vi "CSM - Remove Module in Broadcast Registry.vi"(0 "CSM Name":string, 11 "Error In":errorcluster caption="error in (no error)") -> (4 "CSM Name (Dup)":string, 15 "error out":errorcluster)   [LabVIEW 2017, in "Communicable State Machine.lvlib"]
doc: "### CSM - Remove Module in Broadcast Registry.vi\n\n-- <b>Controls</b> --\n- <b>CSM Name</b>:\n\n-- <b>Indicators</b> --\n- <b>CSM Name(dup)</b>:"
uses:
  _Support/FGV-BroadcastRegistry/Operation-BroadcastRegistry.ctl
  Communicable State Machine.lvlib
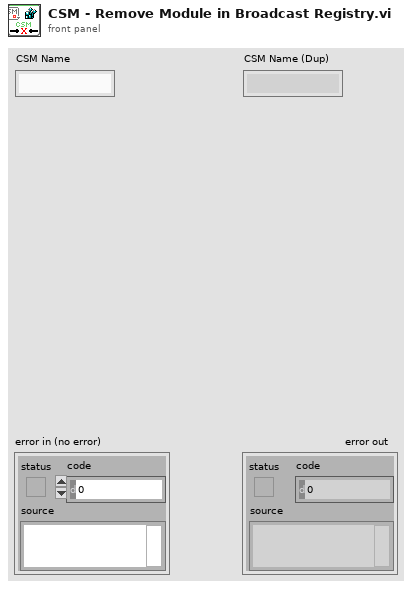
[diagram p1: front panel]
types:
  T1 = typedef "Communicable State Machine.lvlib/Operation-BroadcastRegistry.ctl" = enum16{"Delete Source Module", "Delete Target Module", "Remove Module", "Register", "Unregister", "Check", "List Status", "List Entries", "List Status Of Source", "Drop"}
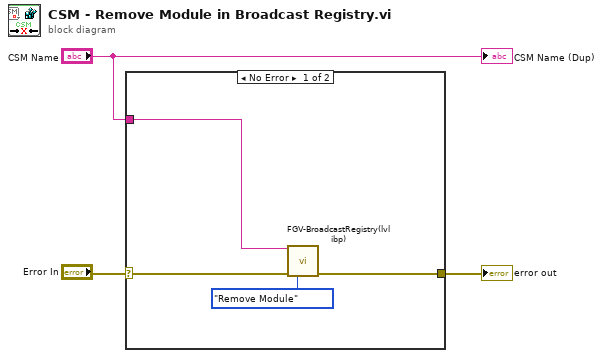
[diagram p0: block diagram]
diagram:
  n1 = case shown="No Error" "Error In" {
    selector: "Error In" -> [w6 w8]
    tunnel: [w5 w8] -> w2
    tunnel: "CSM Name" -> [w4 _]
    frame No Error {
      n2 = call "FGV-BroadcastRegistry(lvlibp).vi"("Source"=w4, "Error In"=w6, "Operation"=Operation-BroadcastRegistry."Remove Module") -> ("error out"=w5:errorcluster)  [unwired: 11 in, 1 out]
    }
    frame Error {
    }
  }
  "error out" <- w2
  "CSM Name (Dup)" <- "CSM Name"
